vi "ReadDhtSensor.vi"(8 "error in (no error)":errorcluster, 9 "DHT Type":T1 items=["DHT11", "DHT22", "DHT21", "AM2301"], 10 "Digital Pin":T2=4 items=["D2"=2, "D3"=3, "D4"=4, "D5"=5, "D6"=6, "D7"=7, "D8"=8, "D9"=9, "A0"=14, "A1"=15, "A2"=16, "A3"=17], 11 "GrovePi in":refnum<class "GrovePi.lvclass">) -> (0 "error out":errorcluster, 1 "Humidity":sgl, 2 "Temperature":sgl, 3 "GrovePi out":refnum<class "GrovePi.lvclass">)   [LabVIEW 2014, in "GrovePi.lvclass"]
doc: "Returns the Temperature and Humidity from a DHT sensor connected to a Digital Pin on the GrovePi."
uses:
  GrovePi.lvclass
  Pin.ctl
  DhtType.ctl
  Command.ctl
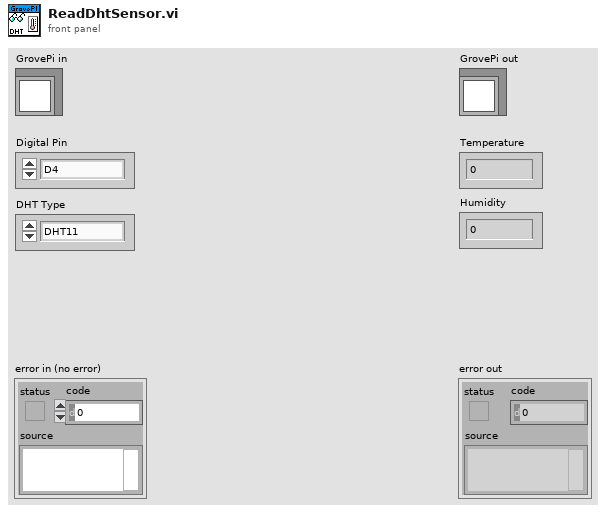
[diagram p1: front panel]
types:
  T1 = typedef "GrovePi.lvclass/DhtType.ctl" = u8
  T2 = typedef "GrovePi.lvclass/Pin.ctl" = u8
  T3 = typedef "GrovePi.lvclass/Command.ctl" = u8
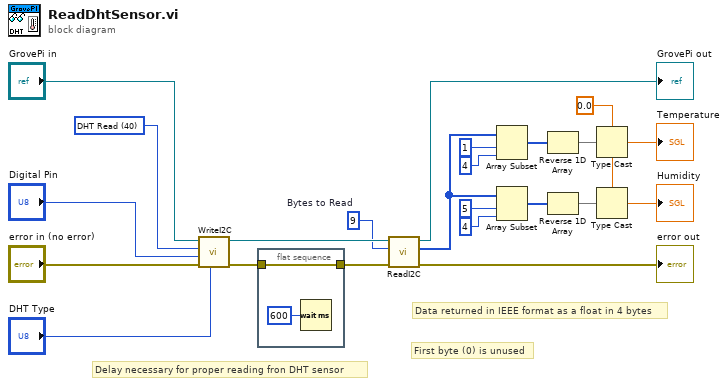
[diagram p0: block diagram]
diagram:
  w3 = sgl 0.0
  w17 = u8 9  # Bytes to Read
  w21 = T3 40 items=["Digital Read"=1, "Digital Write"=2, "Analog Read"=3, "Analog Write"=4, "Pin Mode"=5, "Ultrasonic Read"=7, "Version"=8, "Dust Sensor Read"=10, "Encoder Read"=11, "Flow Read"=12, "Flow Disabled"=13, "Dust Sensor Enable"=14, "Dust Sensor Disable"=15, "Encoder Enable"=16, "Encoder Disable"=17, "Flow Enable"=18, "Accelerometer Read"=20, "RTC Read"=30, "DHT Read"=40] ("Command")
  # "Data returned in IEEE format as a float in 4 bytes"
  # "Delay necessary for proper reading fron DHT sensor"
  # "First byte (0) is unused"
  n1 = call "WriteI2C.vi"("Byte 2"="DHT Type", "error in (no error)"="error in (no error)", "Pin"="Digital Pin", "Command"=w21, "GrovePi in"="GrovePi in") -> ("error out"=w20:errorcluster, "GrovePi out"=w18:refnum<class "GrovePi.lvclass">)  [unwired: 4 in, 1 out]
  n2 = flat-sequence {
    tunnel: w20 -> [w24]
    tunnel: [w24] -> w19
    frame #0 {
      n3 = Wait (ms)(milliseconds to wait=u32 600) -> ()  [unwired: 1 out]
    }
  }
  n4 = call "ReadI2C.vi"("error in (no error)"=w19, "Bytes to Read"=w17, "GrovePi in"=w18) -> ("error out"=→"error out":errorcluster, "Message"=w8:u8[], "GrovePi out"=→"GrovePi out":refnum<class "GrovePi.lvclass">)  [unwired: 6 in]
  n5 = Array Subset(array=w8, index=1, length=4) -> (w7:u8[])
  n6 = Array Subset(array=w8, index=5, length=4) -> (w4:u8[])
  n7 = Reverse 1D Array(array=w7) -> (reversed array=w2:u8[])
  n8 = Reverse 1D Array(array=w4) -> (reversed array=w1:u8[])
  n9 = Type Cast(type=w3, x=w2) -> (*(type *) &x=→"Temperature":sgl)
  n10 = Type Cast(type=w3, x=w1) -> (*(type *) &x=→"Humidity":sgl)
